vi "CronTab@CronStart__Parameter.vi"(1 "ParamterIn":string) -> (0 "ParamterOut":string)   [LabVIEW 2020]
panel:
  in  "Conditioin":string(combo)
  in  "Month":string(combo)="*"
  in  "Day":string(combo)="/5"
  in  "Week":string(combo)="Sun"
  in  "Hour":string(combo)="*"
  in  "Min":string(combo)="/5"
  in  "Sec":string(combo)="/5"
  in  "CronTabName":string(combo)
  in  "Confirm":bool
  # "CronTab@CronStart $CronTabName, $Sec $Min $Hour $Week $Day $Mon"
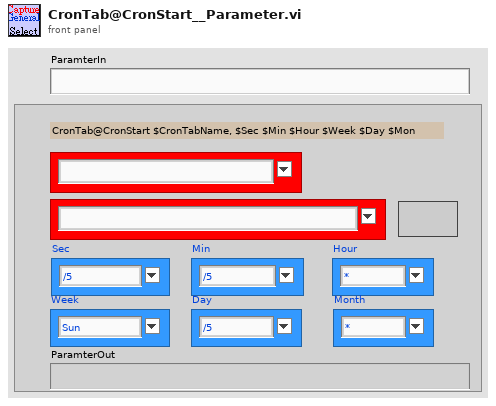
[diagram p1: front panel]
types:
  T1 = enum16{"Init", "Add", "Enable", "Disable", "Get"}
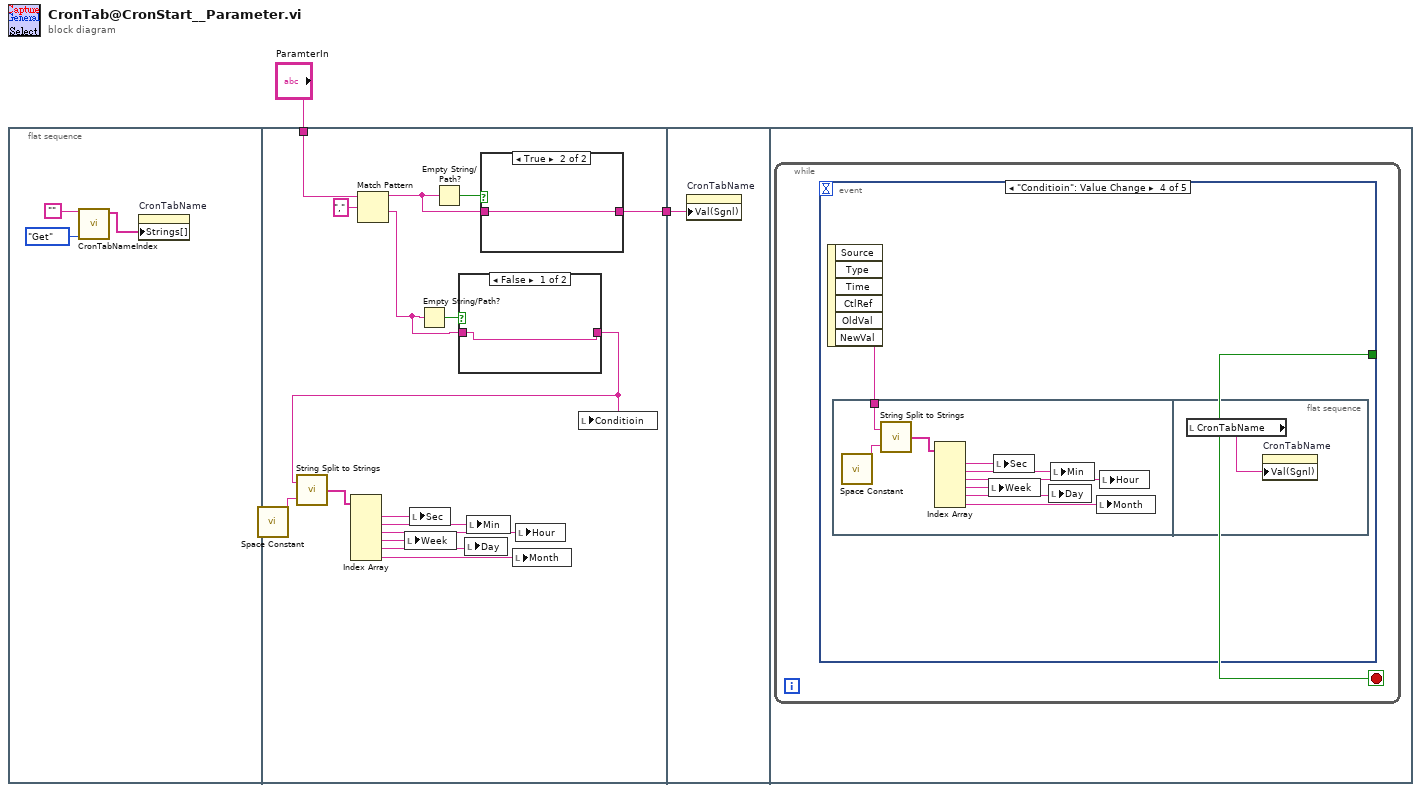
[diagram p0: block diagram]
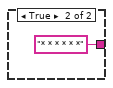
[diagram p2: hidden frame]
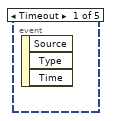
[diagram p4: hidden frame]
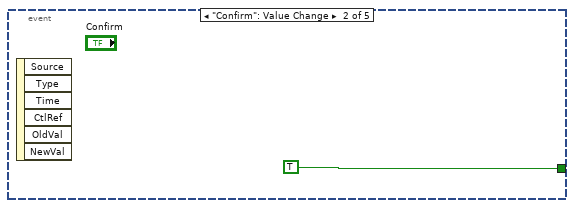
[diagram p5: hidden frame]
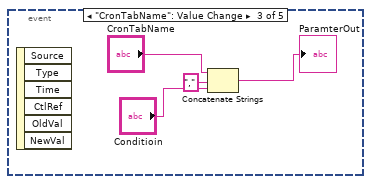
[diagram p6: hidden frame]
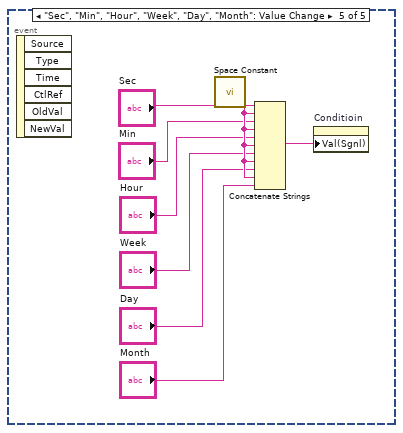
[diagram p7: hidden frame]
diagram:
  n1 = flat-sequence {
    tunnel: "ParamterIn" -> [w19]
    tunnel: [w20] -> w1
    tunnel: w1 -> [w26]
    frame #0 {
      n2 = call "CronTabNameIndex.vi"("OP"=T1."Get", "CronTabName"="") -> ("CronTabNameS"=w3:string[])  [unwired: 6 in, 3 out]
      n3 = property on="CronTabName" class="CmbBox"("Strings[]"=w3) -> ()  [unwired: 2 in, 2 out]
    }
    frame #1 {
      n4 = call <vilib>:"Space Constant.vi"() -> ("String"=w6:string)
      n5 = Match Pattern(string=w19, regular expression=",") -> (before substring=w16:string, after substring=w14:string)  [unwired: 1 in, 2 out]
      n6 = Empty String/Path?(string/path=w14) -> (empty?=w15:bool)
      n7 = Empty String/Path?(string/path=w16) -> (empty?=w21:bool)
      n8 = case shown="False" w15 {
        tunnel: w14 -> [w22 _]
        tunnel: [w22 "* * * * * *" ("ParamterIn")] -> w13
        frame False {
        }
        frame True {
        }
      }
      n9 = call "String Split to Strings.vi"("search string/char (-)"=w6, "String"=w13) -> ("Array"=w17:string[])
      n10 = Index Array(array=w17) -> (element #1=w12:string, element #2=w11:string, element #3=w10:string, element #4=w9:string, element #5=w8:string, element #6=w7:string)  [unwired: 6 in]
      n11 = local write "Week"(w9) -> ()
      n12 = local write "Sec"(w12) -> ()
      n13 = local write "Day"(w8) -> ()
      n14 = local write "Min"(w11) -> ()
      n15 = case shown="True" w21 {
        tunnel: w16 -> [w24 w25]
        tunnel: [w24 w25] -> w20
        frame False {
        }
        frame True {
        }
      }
      n16 = local write "Month"(w7) -> ()
      n17 = local write "Hour"(w10) -> ()
      n18 = local write "Conditioin"(w13) -> ()
    }
    frame #2 {
      n19 = property on="CronTabName" class="CmbBox"("Val(Sgnl)"=w26) -> ()  [unwired: 2 in, 2 out]
    }
    frame #3 {
      n20 = while {
        stop <- w27 stop-if-true
        n21 = event shown="[3] \"Conditioin\": Value Change" {
          selector: _ -> [_ _ _ _ _]
          dyn-events: _ -> [_ _ _ _ _]
          timeout: _ -> [_ _ _ _ _]
          tunnel: [_ TRUE _ _ _] -> w27
          event Timeout {
            n22 = event-data() -> ()  [unwired: 1 in, 3 out]
          }
          event "Confirm": Value Change {
            n23 = event-data() -> ()  [unwired: 1 in, 6 out]
          }
          event "CronTabName": Value Change {
            n24 = event-data() -> ()  [unwired: 1 in, 6 out]
            n25 = Concatenate Strings("CronTabName", "," ("string"), "Conditioin") -> (→"ParamterOut":string)
          }
          event "Conditioin": Value Change {
            n26 = event-data() -> ("NewVal"=w33:string)  [unwired: 1 in, 5 out]
            n27 = flat-sequence {
              tunnel: w33 -> [w34]
              frame #0 {
                n28 = call <vilib>:"Space Constant.vi"() -> ("String"=w42:string)
                n29 = call "String Split to Strings.vi"("search string/char (-)"=w42, "String"=w34) -> ("Array"=w35:string[])
                n30 = Index Array(array=w35) -> (element #1=w36:string, element #2=w37:string, element #3=w38:string, element #4=w39:string, element #5=w40:string, element #6=w41:string)  [unwired: 6 in]
                n31 = local write "Week"(w39) -> ()
                n32 = local write "Sec"(w36) -> ()
                n33 = local write "Day"(w40) -> ()
                n34 = local write "Min"(w37) -> ()
                n35 = local write "Month"(w41) -> ()
                n36 = local write "Hour"(w38) -> ()
              }
              frame #1 {
                n37 = local read "CronTabName"() -> (w43:string)
                n38 = property on="CronTabName" class="CmbBox"("Val(Sgnl)"=w43) -> ()  [unwired: 2 in, 2 out]
              }
            }
          }
          event "Sec", "Min", "Hour", "Week", "Day", "Month": Value Change {
            n39 = event-data() -> ()  [unwired: 1 in, 6 out]
            n40 = call <vilib>:"Space Constant.vi"() -> ("String"=w50:string)
            n41 = Concatenate Strings("Sec", w50, "Min", w50, "Hour", w50, "Week", w50, "Day", w50, "Month") -> (w44:string)
            n42 = property on="Conditioin" class="CmbBox"("Val(Sgnl)"=w44) -> ()  [unwired: 2 in, 2 out]
          }
        }
      }
    }
  }
